vi "Find All Minima 1D.vi"(4 "formula":string, 5 "accuracy":dbl=1e-08 format="%.2e", 6 "end":dbl=1.0 format="%.2f", 7 "start":dbl format="%.2f", 8 "algorithm":u16(ring) items=["Golden Section Search", "Brent with Derivatives"], 9 "step type":u16(ring) items=["fixed function", "modified function"]) -> (0 "error":i32, 1 "ticks":u32, 2 "f(Minima)":dbl[](array[numeric]) format="%.2f", 3 "Minima":dbl[](array[numeric]) format="%.2f")   [LabVIEW 2014, in "NI_Gmath.lvlib"]
doc: "Determines all local minima of a given function in a given interval."
uses:
  NI_Gmath.lvlib
panel:
  # "Example:\n\n accuracy: 1E-8 \n step type: fixed function\n algorithm: Golden Section Search  \n start: 0.0\n end: 1.0\n formula: x^2+sin(x-1)^2"
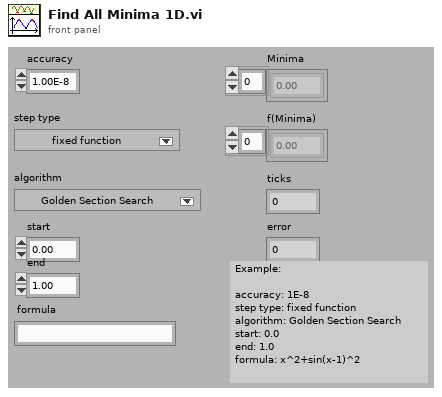
[diagram p1: front panel]
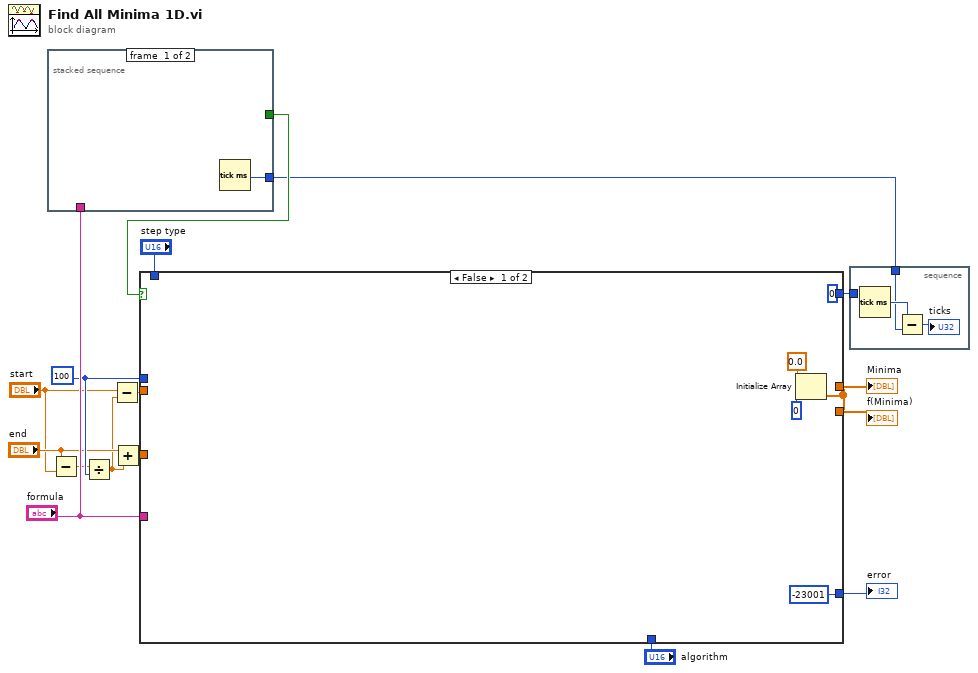
[diagram p0: block diagram]
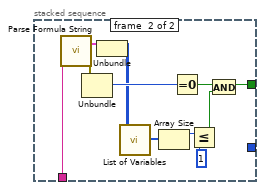
[diagram p2: hidden frame]
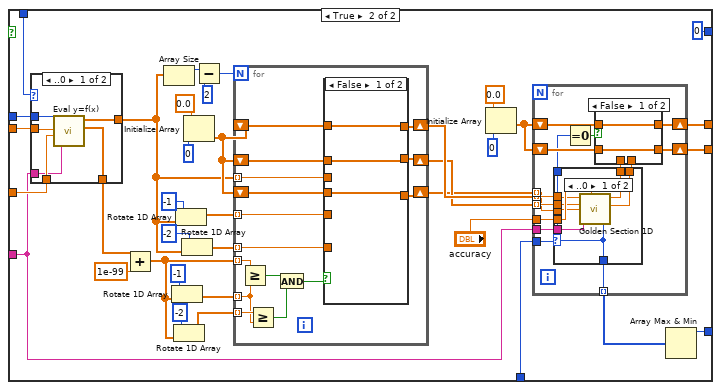
[diagram p3: hidden frame]
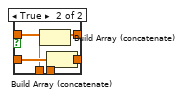
[diagram p4: hidden frame]
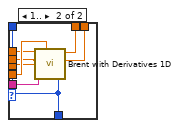
[diagram p5: hidden frame]
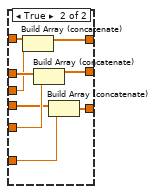
[diagram p6: hidden frame]
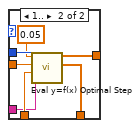
[diagram p7: hidden frame]
diagram:
  w7 = u32 100
  n1 = stacked-sequence {
    tunnel: [_ w28] -> w16
    tunnel: [w17 _] -> w15
    tunnel: "formula" -> [_ w20]
    frame #0 {
      n2 = Tick Count (ms)() -> (millisecond timer value=w17:u32)
    }
    frame #1 {
      n3 = call "Parse Formula String.vi"("formula"=w20) -> ("error out"=w22:errorcluster, "Parsed Formula"=w19:cluster{"Table":i32[][], "Y Values":dbl[]})  [unwired: 1 in]
      n4 = Unbundle(w22) -> ("code"=w21:i32)  [unwired: 2 out]
      n5 = Unbundle(w19) -> ("Table"=w18:i32[][])  [unwired: 1 out]
      n6 = call "List of Variables.vi"("Table"=w18) -> ("List of variables"=w23:i32[])
      n7 = Array Size(array=w23) -> (size(s)=w24:i32)
      n8 = Equal To 0?(x=w21) -> (x = 0?=w27:bool)
      n9 = Less Or Equal?(x=w24, y=1) -> (x <= y?=w26:bool)
      n10 = And(x=w27, y=w26) -> (x .and. y?=w28:bool)
    }
  }
  n11 = Subtract(x="end", y="start") -> (x-y=w6:dbl)
  n12 = Divide(x=w6, y=w7) -> (x/y=w2:dbl)
  n13 = Subtract(x="start", y=w2) -> (x-y=w1:dbl)
  n14 = Add(x="end", y=w2) -> (x+y=w4:dbl)
  n15 = case shown="False" w16 {
    tunnel: "step type" -> [_ w69]
    tunnel: "formula" -> [_ w58]
    tunnel: w1 -> [_ w68]
    tunnel: w4 -> [_ w67]
    tunnel: [0 0] -> w13
    tunnel: "algorithm" -> [_ w41]
    tunnel: [w30 w36] -> w8
    tunnel: [w30 w37] -> w9
    tunnel: [-23001 w35] -> w10
    tunnel: w7 -> [_ w34]
    frame False {
      n16 = Initialize Array(0.0, 0) -> (w30:dbl[])
    }
    frame True {
      n17 = case shown="..0" w69 {
        tunnel: w34 -> [w141 w146]
        tunnel: w58 -> [w138 w142]
        tunnel: w68 -> [w140 w145]
        tunnel: w67 -> [w139 w143]
        tunnel: [w136 w148] -> w38
        tunnel: [w137 w147] -> w39
        frame ..0 {
          n18 = call "Eval y=f(x).vi"("formula"=w138, "end"=w139, "start"=w140, "number of points"=w141) -> ("Y Values"=w136:dbl[], "X Values"=w137:dbl[])  [unwired: 2 out]
        }
        frame 1.. {
          n19 = call "Eval y=f(x) Optimal Step.vi"("number of points"=w146, "formula"=w142, "end"=w143, "start"=w145, "epsilon"=0.05) -> ("Y Values"=w148:dbl[], "X Values"=w147:dbl[])  [unwired: 2 out]
        }
      }
      n20 = Add(x=w38, y=1e-99) -> (x+y=w45:dbl[])
      n21 = Array Size(array=w39) -> (size(s)=w49:i32)
      n22 = Rotate 1D Array(1:w45, 2:-1) -> (0:w65:dbl[])
      n23 = Rotate 1D Array(1:w45, 2:-2) -> (0:w44:dbl[])
      n24 = Rotate 1D Array(1:w39, 2:-1) -> (0:w60:dbl[])
      n25 = Rotate 1D Array(1:w39, 2:-2) -> (0:w50:dbl[])
      n26 = Initialize Array(0.0, 0) -> (w52:dbl[])
      n27 = Subtract(x=w49, y=2) -> (x-y=w48:i32)
      n28 = for {
        N: w48 -> [_]
        tunnel: w45 -> [w114] mode=indexing
        tunnel: w65 -> [w109] mode=indexing
        shift-right: [w122] -> w59
        shift-left: w52 -> [w123]
        shift-right: [w120] -> w53
        shift-left: w52 -> [w121]
        tunnel: w39 -> [w119] mode=indexing
        tunnel: w60 -> [w118] mode=indexing
        shift-right: [w116] -> w43
        shift-left: w52 -> [w117]
        tunnel: w50 -> [w115] mode=indexing
        tunnel: w44 -> [w113] mode=indexing
        n29 = Greater Or Equal?(x=w114, y=w109) -> (x >= y?=w112:bool)
        n30 = Greater Or Equal?(x=w113, y=w109) -> (x >= y?=w111:bool)
        n31 = And(x=w112, y=w111) -> (x .and. y?=w110:bool)
        n32 = case shown="False" w110 {
          tunnel: w123 -> [w126 w135]
          tunnel: [w126 w134] -> w122
          tunnel: w121 -> [w125 w133]
          tunnel: [w125 w132] -> w120
          tunnel: w119 -> [_ w131]
          tunnel: w118 -> [_ w130]
          tunnel: w117 -> [w124 w129]
          tunnel: [w124 w128] -> w116
          tunnel: w115 -> [_ w127]
          frame False {
          }
          frame True {
            n33 = Build Array (concatenate)(w135, w131) -> (w134:dbl[])
            n34 = Build Array (concatenate)(w133, w130) -> (w132:dbl[])
            n35 = Build Array (concatenate)(w129, w127) -> (w128:dbl[])
          }
        }
      }
      n36 = Initialize Array(0.0, 0) -> (w54:dbl[])
      n37 = for {
        tunnel: w59 -> [w78] mode=indexing
        tunnel: w53 -> [w77] mode=indexing
        tunnel: w58 -> [w79]
        shift-right: [w80] -> w37
        shift-left: w54 -> [w84]
        shift-right: [w73] -> w36
        shift-left: w54 -> [w82]
        tunnel: w43 -> [w76] mode=indexing
        tunnel: "accuracy" -> [w75]
        tunnel: w41 -> [w74]
        tunnel: [w72] -> w40 mode=indexing
        n38 = case shown="..0" w74 {
          tunnel: w75 -> [w98 w105]
          tunnel: w76 -> [w94 w102]
          tunnel: w77 -> [w95 w103]
          tunnel: w78 -> [w96 w104]
          tunnel: w79 -> [w97 w106]
          tunnel: [w100 w108] -> w81
          tunnel: [w99 w107] -> w83
          tunnel: [w93 w101] -> w72
          tunnel: [w93 w101] -> w71
          frame ..0 {
            n39 = call "Golden Section 1D.vi"("accuracy"=w98, "formula"=w97, "c (start)"=w94, "b (start)"=w95, "a (start)"=w96) -> ("error"=w93:i32, "f(minimum)"=w100:dbl, "minimum"=w99:dbl)  [unwired: 1 out]
          }
          frame 1.. {
            n40 = call "Brent with Derivatives 1D.vi"("accuracy"=w105, "formula"=w106, "c (start)"=w102, "b (start)"=w103, "a (start)"=w104) -> ("error"=w101:i32, "f(minimum)"=w108:dbl, "minimum"=w107:dbl)  [unwired: 1 out]
          }
        }
        n41 = Equal To 0?(x=w71) -> (x = 0?=w70:bool)
        n42 = case shown="False" w70 {
          tunnel: [w85 w92] -> w73
          tunnel: [w86 w91] -> w80
          tunnel: w81 -> [_ w90]
          tunnel: w82 -> [w85 w89]
          tunnel: w83 -> [_ w88]
          tunnel: w84 -> [w86 w87]
          frame False {
          }
          frame True {
            n43 = Build Array (concatenate)(w87, w88) -> (w91:dbl[])
            n44 = Build Array (concatenate)(w89, w90) -> (w92:dbl[])
          }
        }
      }
      n45 = Array Max & Min(array=w40) -> (max value=w35:i32)  [unwired: 3 out]
    }
  }
  "f(Minima)" <- w8
  "Minima" <- w9
  "error" <- w10
  n46 = stacked-sequence {
    tunnel: w15 -> [w149]
    tunnel: w13 -> [_]
    frame #0 {
      n47 = Tick Count (ms)() -> (millisecond timer value=w150:u32)
      n48 = Subtract(x=w150, y=w149) -> (x-y=→"ticks":u32)
    }
  }
